vi "SP_OEE_2_test.vi"() -> ()   [LabVIEW 2017] (continued)
                      tunnel: [w17350] -> w17056
                      tunnel: [w17349] -> w17055
                      tunnel: [w17348] -> w17054
                      tunnel: [w17347] -> w17053
                      tunnel: [w17346] -> w17052
                      tunnel: [w17345] -> w17051
                      tunnel: [w17343] -> w17050
                      tunnel: [w17341] -> w17049
                      tunnel: [w17337] -> w17048
                      tunnel: [w17335] -> w17047
                      tunnel: w17062 -> [w17336]
                      tunnel: w17061 -> [w17332]
                      tunnel: [w17331] -> w17046
                      tunnel: w17060 -> [w17331]
                      tunnel: w17019 -> [w17329]
                      tunnel: w17059 -> [w17380]
                      tunnel: w17058 -> [w17373]
                      tunnel: w17057 -> [w17364]
                      tunnel: w17056 -> [w17372]
                      tunnel: w17055 -> [w17362]
                      tunnel: w17054 -> [w17371]
                      tunnel: w17053 -> [w17360]
                      tunnel: w17052 -> [w17370]
                      tunnel: w17051 -> [w17358]
                      tunnel: w17050 -> [w17394]
                      tunnel: w17049 -> [w17393]
                      tunnel: w17048 -> [w17369]
                      tunnel: w17047 -> [w17356]
                      tunnel: [w17394] -> w17045
                      tunnel: [w17393] -> w17044
                      tunnel: [w17387] -> w17043
                      tunnel: [w17380] -> w17042
                      tunnel: [w17379] -> w17041
                      tunnel: [w17378] -> w17040
                      tunnel: [w17377] -> w17039
                      tunnel: [w17376] -> w17038
                      tunnel: [w17375] -> w17037
                      tunnel: [w17374] -> w17036
                      tunnel: [w17373] -> w17035
                      tunnel: [w17372] -> w17034
                      tunnel: [w17371] -> w17033
                      tunnel: [w17370] -> w17032
                      tunnel: [w17369] -> w17031
                      tunnel: [w17354] -> w17030
                      tunnel: w17046 -> [w17354]
                      tunnel: [w17407] -> _
                      tunnel: [w17403] -> _
                      tunnel: w17045 -> [w17404]
                      tunnel: w17044 -> [w17407]
                      tunnel: w17043 -> [w17398]
                      tunnel: w17042 -> [w17405]
                      tunnel: w17041 -> [_]
                      tunnel: w17040 -> [_]
                      tunnel: w17039 -> [_]
                      tunnel: w17038 -> [_]
                      tunnel: w17037 -> [w17397]
                      tunnel: w17036 -> [w17399]
                      tunnel: w17035 -> [_]
                      tunnel: w17034 -> [_]
                      tunnel: w17033 -> [_]
                      tunnel: w17032 -> [_]
                      tunnel: w17031 -> [w17396]
                      tunnel: w17030 -> [w17402]
                      frame #0 {
                        w17134 = "%Y-%m-%d" ("time format string (%c)")
                        n3102 = Decimal String To Number(string=w17120) -> (number=w17121:i32)  [unwired: 2 in, 1 out]
                        n3103 = property on="Table" class="Tbl (strict)"("Visible"=TRUE) -> ()  [unwired: 2 in, 2 out]
                        n3104 = Format Date/Time String(time format string (%c)=w17134, seconds (now)=w17126) -> (date/time string=w17135:string)  [unwired: 1 in]
                        n3105 = Format Date/Time String(time format string (%c)=w17134, seconds (now)=w17125) -> (date/time string=w17133:string)  [unwired: 1 in]
                        n3106 = Format Into String(format string="Where BREAKDOWN_DATE between '%s' and '%s' and  SHIFT_ID = '%d'  ", w17135, w17133, w17121) -> (resulting string=w17132:string)  [unwired: 2 in, 1 out]
                        n3107 = call <vilib>:"DB Tools Select Data.vi"("condition"=w17132, "error in (no error)"=w17141, "columns"=string[] ["BREAKDOWN_DATE"], "table"="STATION_1_LOG_HISTORY", "connection reference"=w17143) -> ("error out"=w17128:errorcluster, "data"=w17131:variant[][], "connection reference out"=w17142:T2)  [unwired: 1 in]
                        n3108 = property on="Table 2" class="Tbl (strict)"("Visible"=FALSE) -> ()  [unwired: 2 in, 2 out]
                        n3109 = xnode "Database Variant To Data"("database variant"=w17131, "error in (no error)"=w17128, "type"=string[][] [] ("Elements Found")) -> ("data"=w17129:string[][], "error out"=w17127:errorcluster)
                        n3110 = Index Array(array=w17129, index (col)=0 ("disabled index (col)")) -> (element=w17137:string[])  [unwired: 1 in]
                        n3111 = call "Search_1d_array_element.vi"("Count in"=string[] [] ("Elements Found"), "BD Date"=w17137, "Elements Found in"=string[] [] ("Elements Found")) -> ("Elements Found out"=w17124:string[])  [unwired: 4 in, 2 out]
                        n3112 = Build Array(w17124) -> (w17147:string[][])
                        n3113 = Transpose 2D Array(2D array=w17147) -> (transposed array=w17146:string[][])
                      }
                      frame #1 {
                        n3114 = disable-structure shown="Enabled" {
                          disable-tunnel: w17209 -> [w17220 w17222]
                          disable-tunnel: [w17219 w17222] -> w17208
                          disable-tunnel: w17207 -> [w17218 w17223]
                          disable-tunnel: [w17217 w17223] -> w17206
                          disable-tunnel: w17204 -> [w17215 _]
                          disable-tunnel: w17203 -> [w17214 _]
                          disable-tunnel: [w17213 _] -> w17202
                          disable-tunnel: [w17212 _] -> w17199
                          disable-tunnel: w17197 -> [w17211 _]
                          disable-tunnel: w17194 -> [w17210 w17221]
                          disable-tunnel: [_ w17221] -> w17193
                          frame Disabled {
                            n3115 = call "Stack_holderwise_total_bd_count_&_duration_2.vi"("Refnum in"=w17220, "BREAKDOWN_STK_HOLD_ID"=1, "condition"=w17211, "Form Date"=w17215, "To Date"=w17214, "error in (no error)"=w17218, "Shift"=w17210) -> ("Refnum out"=w17219:T2, "Count out"=w17213:string[], "appended array"=w17212:dbl[], "error out"=w17217:errorcluster)  [unwired: 5 in]
                          }
                          frame Enabled {
                          }
                        }
                        n3116 = call "NUMERIC TO STRING.vi"("appended array"=w17199) -> ("Array"=w17198:string[])  [unwired: 4 in]
                        n3117 = call "Insert_empty_element_with_zero.vi"("searched date"=w17202, "fixed date"=w17200) -> ("O/P"=w17195:string[])  [unwired: 9 in]
                        n3118 = call "Insert_empty_element_with_zero.vi"("searched date"=w17198, "fixed date"=w17200) -> ("O/P"=w17201:string[])  [unwired: 9 in]
                      }
                      frame #2 {
                        n3119 = disable-structure shown="Enabled" {
                          disable-tunnel: w17239 -> [w17253 w17255]
                          disable-tunnel: [w17252 w17255] -> w17238
                          disable-tunnel: w17237 -> [w17251 w17256]
                          disable-tunnel: [w17250 w17256] -> w17236
                          disable-tunnel: w17235 -> [w17249 _]
                          disable-tunnel: w17234 -> [w17248 _]
                          disable-tunnel: [w17247 _] -> w17233
                          disable-tunnel: [w17246 _] -> w17229
                          disable-tunnel: w17227 -> [w17245 _]
                          disable-tunnel: w17225 -> [w17243 w17254]
                          disable-tunnel: [_ w17254] -> w17224
                          frame Disabled {
                            n3120 = call "Stack_holderwise_total_bd_count_&_duration_2.vi"("Refnum in"=w17251, "BREAKDOWN_STK_HOLD_ID"=2, "condition"=w17245, "Form Date"=w17249, "To Date"=w17248, "error in (no error)"=w17253, "Shift"=w17243) -> ("Refnum out"=w17250:T2, "Count out"=w17247:string[], "appended array"=w17246:dbl[], "error out"=w17252:errorcluster)  [unwired: 5 in]
                          }
                          frame Enabled {
                          }
                        }
                        n3121 = call "Insert_empty_element_with_zero.vi"("searched date"=w17233, "fixed date"=w17230) -> ("O/P"=w17232:string[])  [unwired: 9 in]
                        n3122 = call "NUMERIC TO STRING.vi"("appended array"=w17229) -> ("Array"=w17228:string[])  [unwired: 4 in]
                        n3123 = call "Insert_empty_element_with_zero.vi"("searched date"=w17228, "fixed date"=w17230) -> ("O/P"=w17231:string[])  [unwired: 9 in]
                      }
                      frame #3 {
                        n3124 = disable-structure shown="Enabled" {
                          disable-tunnel: w17272 -> [w17288 w17290]
                          disable-tunnel: [w17287 w17290] -> w17271
                          disable-tunnel: w17270 -> [w17286 w17291]
                          disable-tunnel: [w17285 w17291] -> w17269
                          disable-tunnel: w17268 -> [w17284 _]
                          disable-tunnel: w17267 -> [w17283 _]
                          disable-tunnel: [w17282 _] -> w17266
                          disable-tunnel: [w17281 _] -> w17262
                          disable-tunnel: w17260 -> [w17280 _]
                          disable-tunnel: w17258 -> [w17278 w17289]
                          disable-tunnel: [_ w17289] -> w17257
                          frame Disabled {
                            n3125 = call "Stack_holderwise_total_bd_count_&_duration_2.vi"("Refnum in"=w17286, "BREAKDOWN_STK_HOLD_ID"=3, "condition"=w17280, "Form Date"=w17284, "To Date"=w17283, "error in (no error)"=w17288, "Shift"=w17278) -> ("Refnum out"=w17285:T2, "Count out"=w17282:string[], "appended array"=w17281:dbl[], "error out"=w17287:errorcluster)  [unwired: 5 in]
                          }
                          frame Enabled {
                          }
                        }
                        n3126 = call "Insert_empty_element_with_zero.vi"("searched date"=w17266, "fixed date"=w17263) -> ("O/P"=w17265:string[])  [unwired: 9 in]
                        n3127 = call "NUMERIC TO STRING.vi"("appended array"=w17262) -> ("Array"=w17261:string[])  [unwired: 4 in]
                        n3128 = call "Insert_empty_element_with_zero.vi"("searched date"=w17261, "fixed date"=w17263) -> ("O/P"=w17264:string[])  [unwired: 9 in]
                      }
                      frame #4 {
                        n3129 = disable-structure shown="Enabled" {
                          disable-tunnel: w17307 -> [w17325 w17328]
                          disable-tunnel: w17306 -> [w17324 w17327]
                          disable-tunnel: [w17323 w17327] -> w17305
                          disable-tunnel: [w17322 w17328] -> w17304
                          disable-tunnel: w17303 -> [w17321 _]
                          disable-tunnel: w17302 -> [w17320 _]
                          disable-tunnel: [w17319 _] -> w17301
                          disable-tunnel: [w17318 _] -> w17297
                          disable-tunnel: w17295 -> [w17317 _]
                          disable-tunnel: w17293 -> [w17315 w17326]
                          disable-tunnel: [_ w17326] -> w17292
                          frame Disabled {
                            n3130 = call "Stack_holderwise_total_bd_count_&_duration_2.vi"("Refnum in"=w17324, "BREAKDOWN_STK_HOLD_ID"=4, "condition"=w17317, "Form Date"=w17321, "To Date"=w17320, "error in (no error)"=w17325, "Shift"=w17315) -> ("Refnum out"=w17323:T2, "Count out"=w17319:string[], "appended array"=w17318:dbl[], "error out"=w17322:errorcluster)  [unwired: 5 in]
                          }
                          frame Enabled {
                          }
                        }
                        n3131 = call "Insert_empty_element_with_zero.vi"("searched date"=w17301, "fixed date"=w17298) -> ("O/P"=w17300:string[])  [unwired: 9 in]
                        n3132 = call "NUMERIC TO STRING.vi"("appended array"=w17297) -> ("Array"=w17296:string[])  [unwired: 4 in]
                        n3133 = call "Insert_empty_element_with_zero.vi"("searched date"=w17296, "fixed date"=w17298) -> ("O/P"=w17299:string[])  [unwired: 9 in]
                      }
                      frame #5 {
                        n3134 = call "Stack_holderwise_total_bd_count_&_duration_2.vi"("Refnum in"=w17342, "BREAKDOWN_STK_HOLD_ID"=5, "condition"=w17332, "Form Date"=w17339, "To Date"=w17340, "error in (no error)"=w17344, "Shift"=w17329) -> ("Refnum out"=w17341:T2, "Count out"=w17338:string[], "appended array"=w17334:dbl[], "error out"=w17343:errorcluster)  [unwired: 5 in]
                        n3135 = call "NUMERIC TO STRING.vi"("appended array"=w17334) -> ("Array"=w17333:string[])  [unwired: 4 in]
                        n3136 = call "Insert_empty_element_with_zero.vi"("searched date"=w17338, "fixed date"=w17336) -> ("O/P"=w17337:string[])  [unwired: 9 in]
                        n3137 = call "Insert_empty_element_with_zero.vi"("searched date"=w17333, "fixed date"=w17336) -> ("O/P"=w17335:string[])  [unwired: 9 in]
                      }
                      frame #6 {
                        n3138 = call "String to numeric.vi"("Array"=w17364) -> ("Array 2"=w17363:dbl[])  [unwired: 4 in]
                        n3139 = call "String to numeric.vi"("Array"=w17362) -> ("Array 2"=w17361:dbl[])  [unwired: 4 in]
                        n3140 = call "String to numeric.vi"("Array"=w17360) -> ("Array 2"=w17359:dbl[])  [unwired: 4 in]
                        n3141 = call "String to numeric.vi"("Array"=w17358) -> ("Array 2"=w17357:dbl[])  [unwired: 4 in]
                        n3142 = call "String to numeric.vi"("Array"=w17356) -> ("Array 2"=w17355:dbl[])  [unwired: 4 in]
                        n3143 = Decimal String To Number(string=w17369) -> (number=w17388:i32[])  [unwired: 2 in, 1 out]
                        n3144 = Decimal String To Number(string=w17370) -> (number=w17389:i32[])  [unwired: 2 in, 1 out]
                        n3145 = Decimal String To Number(string=w17371) -> (number=w17390:i32[])  [unwired: 2 in, 1 out]
                        n3146 = Decimal String To Number(string=w17372) -> (number=w17391:i32[])  [unwired: 2 in, 1 out]
                        n3147 = Decimal String To Number(string=w17373) -> (number=w17386:i32[])  [unwired: 2 in, 1 out]
                        n3148 = Compound Arithmetic op=ADD(w17363, w17361, w17359, w17357, w17355) -> (w17366:dbl[])
                        n3149 = Build Array(w17364) -> (w17385:string[][])
                        n3150 = Build Array(w17362) -> (w17384:string[][])
                        n3151 = Build Array(w17360) -> (w17383:string[][])
                        n3152 = Build Array(w17358) -> (w17382:string[][])
                        n3153 = Build Array(w17356) -> (w17381:string[][])
                        n3154 = Number To Fractional String(number=w17366, precision (6)=i16 2) -> (F-format string=w17365:string[])  [unwired: 2 in]
                        n3155 = Compound Arithmetic op=ADD(w17388, w17389, w17390, w17391, w17386) -> (w17392:i32[])
                        n3156 = Transpose 2D Array(2D array=w17385) -> (transposed array=w17379:string[][])
                        n3157 = Transpose 2D Array(2D array=w17384) -> (transposed array=w17378:string[][])
                        n3158 = Transpose 2D Array(2D array=w17383) -> (transposed array=w17377:string[][])
                        n3159 = Transpose 2D Array(2D array=w17382) -> (transposed array=w17376:string[][])
                        n3160 = Transpose 2D Array(2D array=w17381) -> (transposed array=w17375:string[][])
                        n3161 = Number To Decimal String(number=w17392) -> (decimal integer string=w17387:string[])  [unwired: 1 in]
                        n3162 = Build Array(w17365) -> (w17368:string[][])
                        n3163 = Transpose 2D Array(2D array=w17368) -> (transposed array=w17374:string[][])
                      }
                      frame #7 {
                        w17395 = string[] [""]
                        n3164 = Insert Into Array(array=w17405, index (col)=1 ("disabled index (col)"), new element #1=w17395, new element #2=w17395, new element #3=w17395, new element #4=w17395, new element #5=w17395, new element #6=w17395, new element #7=w17395, new element #8=w17395, new element #9=w17396, new element #10=w17397, new element #11=w17398, new element #12=w17399) -> (w17401:string[][])  [unwired: 1 in]
                        n3165 = call "flot graph for month n year.vi"("BD Date"=w17402, "error in (no error)"=w17404, "Count total"=w17398) -> ("error out"=w17403:errorcluster, "Run-Time Status"=w17400:cluster{"Array 2":timestamp[], dbl[]})  [unwired: 7 in]
                        n3166 = local write "Run-Time Status"(w17400) -> ()
                        n3167 = local write "Table"(w17401) -> ()
                      }
                    }
                  }
                  frame "1" {
                    n3168 = flat-sequence {
                      tunnel: w17418 -> [w17532]
                      tunnel: w17417 -> [w17530]
                      tunnel: [w17516] -> w17508
                      tunnel: [w17531] -> w17507
                      tunnel: w17416 -> [_]
                      tunnel: [w17535] -> w17506
                      tunnel: [w17515] -> w17505
                      tunnel: [w17514] -> w17504
                      tunnel: [w17513] -> w17503
                      tunnel: w17415 -> [w17515]
                      tunnel: w17414 -> [w17514]
                      tunnel: ["Where BREAKDOWN_DATE between '%s'and '%s' and BREAKDOWN_STK_HOLD_ID ='%d' and  SHIFT_ID = '%d' "] -> w17502
                      tunnel: [w17513] -> w17501
                      tunnel: w17413 -> [w17509]
                      tunnel: [w17509] -> w17412
                      tunnel: w17508 -> [w17596]
                      tunnel: w17507 -> [w17598]
                      tunnel: w17506 -> [w17594]
                      tunnel: w17505 -> [w17593]
                      tunnel: w17504 -> [w17592]
                      tunnel: [w17595] -> w17500
                      tunnel: [w17597] -> w17499
                      tunnel: [w17594] -> w17498
                      tunnel: [w17584] -> w17497
                      tunnel: [w17590] -> w17496
                      tunnel: [w17593] -> w17495
                      tunnel: [w17592] -> w17494
                      tunnel: w17503 -> [w17589]
                      tunnel: [w17589] -> w17493
                      tunnel: w17502 -> [w17586]
                      tunnel: [w17586] -> w17492
                      tunnel: [w17585] -> w17491
                      tunnel: w17501 -> [w17585]
                      tunnel: w17412 -> [w17583]
                      tunnel: [w17582] -> w17411
                      tunnel: w17500 -> [w17628]
                      tunnel: w17499 -> [w17626]
                      tunnel: w17498 -> [w17631]
                      tunnel: w17497 -> [w17630]
                      tunnel: w17496 -> [w17629]
                      tunnel: w17495 -> [w17624]
                      tunnel: w17494 -> [w17623]
                      tunnel: [w17631] -> w17490
                      tunnel: [w17630] -> w17489
                      tunnel: [w17629] -> w17488
                      tunnel: [w17627] -> w17487
                      tunnel: [w17621] -> w17486
                      tunnel: [w17620] -> w17485
                      tunnel: [w17625] -> w17484
                      tunnel: [w17624] -> w17483
                      tunnel: [w17623] -> w17482
                      tunnel: w17493 -> [w17619]
                      tunnel: [w17619] -> w17481
                      tunnel: w17492 -> [w17616]
                      tunnel: [w17616] -> w17480
                      tunnel: [w17615] -> w17479
                      tunnel: w17491 -> [w17615]
                      tunnel: w17411 -> [w17614]
                      tunnel: [w17613] -> w17410
                      tunnel: w17490 -> [w17666]
                      tunnel: w17489 -> [w17665]
                      tunnel: w17488 -> [w17664]
                      tunnel: w17487 -> [w17661]
                      tunnel: w17486 -> [w17663]
                      tunnel: w17485 -> [w17662]
                      tunnel: w17484 -> [w17659]
                      tunnel: w17483 -> [w17657]
                      tunnel: w17482 -> [w17656]
                      tunnel: [w17666] -> w17478
                      tunnel: [w17665] -> w17477
                      tunnel: [w17664] -> w17476
                      tunnel: [w17663] -> w17475
                      tunnel: [w17662] -> w17474
                      tunnel: [w17660] -> w17473
                      tunnel: [w17654] -> w17472
                      tunnel: [w17653] -> w17471
                      tunnel: [w17658] -> w17470
                      tunnel: [w17657] -> w17469
                      tunnel: [w17656] -> w17468
                      tunnel: w17481 -> [w17652]
                      tunnel: [w17652] -> w17467
                      tunnel: w17480 -> [w17649]
                      tunnel: [w17649] -> w17466
                      tunnel: [w17648] -> w17465
                      tunnel: w17479 -> [w17648]
                      tunnel: w17410 -> [w17647]
                      tunnel: [w17646] -> w17409
                      tunnel: w17478 -> [w17703]
                      tunnel: w17477 -> [w17702]
                      tunnel: w17476 -> [w17701]
                      tunnel: w17475 -> [w17700]
                      tunnel: w17474 -> [w17699]
                      tunnel: w17473 -> [w17696]
                      tunnel: w17472 -> [w17698]
                      tunnel: w17471 -> [w17697]
                      tunnel: w17470 -> [w17695]
                      tunnel: w17469 -> [w17692]
                      tunnel: w17468 -> [w17691]
                      tunnel: [w17703] -> w17464
                      tunnel: [w17702] -> w17463
                      tunnel: [w17701] -> w17462
                      tunnel: [w17700] -> w17461
                      tunnel: [w17699] -> w17460
                      tunnel: [w17698] -> w17459
                      tunnel: [w17697] -> w17458
                      tunnel: [w17694] -> w17457
                      tunnel: [w17693] -> w17456
                      tunnel: [w17689] -> w17455
                      tunnel: [w17688] -> w17454
                      tunnel: [w17692] -> w17453
                      tunnel: [w17691] -> w17452
                      tunnel: w17467 -> [w17687]
                      tunnel: [w17687] -> w17451
                      tunnel: w17466 -> [w17684]
                      tunnel: [w17684] -> w17450
                      tunnel: [w17683] -> w17449
                      tunnel: w17465 -> [w17683]
                      tunnel: w17409 -> [w17682]
                      tunnel: [w17681] -> w17408
                      tunnel: w17464 -> [w17742]
                      tunnel: w17463 -> [w17741]
                      tunnel: w17462 -> [w17740]
                      tunnel: w17461 -> [w17739]
                      tunnel: w17460 -> [w17738]
                      tunnel: w17459 -> [w17737]
                      tunnel: w17458 -> [w17736]
                      tunnel: w17457 -> [w17731]
                      tunnel: w17456 -> [w17733]
                      tunnel: w17455 -> [w17735]
                      tunnel: w17454 -> [w17734]
                      tunnel: w17453 -> [w17728]
                      tunnel: w17452 -> [w17729]
                      tunnel: [w17742] -> w17448
                      tunnel: [w17741] -> w17447
                      tunnel: [w17740] -> w17446
                      tunnel: [w17739] -> w17445
                      tunnel: [w17738] -> w17444
                      tunnel: [w17737] -> w17443
                      tunnel: [w17736] -> w17442
                      tunnel: [w17735] -> w17441
                      tunnel: [w17734] -> w17440
                      tunnel: [w17732] -> w17439
                      tunnel: [w17730] -> w17438
                      tunnel: [w17726] -> w17437
                      tunnel: [w17724] -> w17436
                      tunnel: w17451 -> [w17725]
                      tunnel: w17450 -> [w17721]
                      tunnel: [w17720] -> w17435
                      tunnel: w17449 -> [w17720]
                      tunnel: w17408 -> [w17718]
                      tunnel: w17448 -> [w17769]
                      tunnel: w17447 -> [w17762]
                      tunnel: w17446 -> [w17753]
                      tunnel: w17445 -> [w17761]
                      tunnel: w17444 -> [w17751]
                      tunnel: w17443 -> [w17760]
                      tunnel: w17442 -> [w17749]
                      tunnel: w17441 -> [w17759]
                      tunnel: w17440 -> [w17747]
                      tunnel: w17439 -> [w17783]
                      tunnel: w17438 -> [w17782]
                      tunnel: w17437 -> [w17758]
                      tunnel: w17436 -> [w17745]
                      tunnel: [w17783] -> w17434
                      tunnel: [w17782] -> w17433
                      tunnel: [w17776] -> w17432
                      tunnel: [w17769] -> w17431
                      tunnel: [w17768] -> w17430
                      tunnel: [w17767] -> w17429
                      tunnel: [w17766] -> w17428
                      tunnel: [w17765] -> w17427
                      tunnel: [w17764] -> w17426
                      tunnel: [w17763] -> w17425
                      tunnel: [w17762] -> w17424
                      tunnel: [w17761] -> w17423
                      tunnel: [w17760] -> w17422
                      tunnel: [w17759] -> w17421
                      tunnel: [w17758] -> w17420
                      tunnel: [w17743] -> w17419
                      tunnel: w17435 -> [w17743]
                      tunnel: [w17796] -> _
                      tunnel: [w17792] -> _
                      tunnel: w17434 -> [w17793]
                      tunnel: w17433 -> [w17796]
                      tunnel: w17432 -> [w17787]
                      tunnel: w17431 -> [w17794]
                      tunnel: w17430 -> [_]
                      tunnel: w17429 -> [_]
                      tunnel: w17428 -> [_]
                      tunnel: w17427 -> [_]
                      tunnel: w17426 -> [w17786]
                      tunnel: w17425 -> [w17788]
                      tunnel: w17424 -> [_]
                      tunnel: w17423 -> [_]
                      tunnel: w17422 -> [_]
                      tunnel: w17421 -> [_]
                      tunnel: w17420 -> [w17785]
                      tunnel: w17419 -> [w17791]
                      frame #0 {
                        w17523 = "%Y-%m-%d" ("time format string (%c)")
                        n3169 = Decimal String To Number(string=w17509) -> (number=w17510:i32)  [unwired: 2 in, 1 out]
                        n3170 = property on="Table" class="Tbl (strict)"("Visible"=TRUE) -> ()  [unwired: 2 in, 2 out]
                        n3171 = Format Date/Time String(time format string (%c)=w17523, seconds (now)=w17515) -> (date/time string=w17524:string)  [unwired: 1 in]
                        n3172 = Format Date/Time String(time format string (%c)=w17523, seconds (now)=w17514) -> (date/time string=w17522:string)  [unwired: 1 in]
                        n3173 = Format Into String(format string="Where BREAKDOWN_DATE between '%s' and '%s' and  SHIFT_ID = '%d'  ", w17524, w17522, w17510) -> (resulting string=w17521:string)  [unwired: 2 in, 1 out]
                        n3174 = call <vilib>:"DB Tools Select Data.vi"("condition"=w17521, "error in (no error)"=w17530, "columns"=string[] ["BREAKDOWN_DATE"], "table"="STATION_1_LOG_HISTORY", "connection reference"=w17532) -> ("error out"=w17517:errorcluster, "data"=w17520:variant[][], "connection reference out"=w17531:T2)  [unwired: 1 in]
                        n3175 = property on="Table 2" class="Tbl (strict)"("Visible"=FALSE) -> ()  [unwired: 2 in, 2 out]
                        n3176 = xnode "Database Variant To Data"("database variant"=w17520, "error in (no error)"=w17517, "type"=string[][] [] ("Elements Found")) -> ("data"=w17518:string[][], "error out"=w17516:errorcluster)
                        n3177 = Index Array(array=w17518, index (col)=0 ("disabled index (col)")) -> (element=w17526:string[])  [unwired: 1 in]
                        n3178 = call "Search_1d_array_element.vi"("Count in"=string[] [] ("Elements Found"), "BD Date"=w17526, "Elements Found in"=string[] [] ("Elements Found")) -> ("Elements Found out"=w17513:string[])  [unwired: 4 in, 2 out]
                        n3179 = Build Array(w17513) -> (w17536:string[][])
                        n3180 = Transpose 2D Array(2D array=w17536) -> (transposed array=w17535:string[][])
                      }
                      frame #1 {
                        n3181 = disable-structure shown="Enabled" {
                          disable-tunnel: w17598 -> [w17609 w17611]
                          disable-tunnel: [w17608 w17611] -> w17597
                          disable-tunnel: w17596 -> [w17607 w17612]
                          disable-tunnel: [w17606 w17612] -> w17595
                          disable-tunnel: w17593 -> [w17604 _]
                          disable-tunnel: w17592 -> [w17603 _]
                          disable-tunnel: [w17602 _] -> w17591
                          disable-tunnel: [w17601 _] -> w17588
                          disable-tunnel: w17586 -> [w17600 _]
                          disable-tunnel: w17583 -> [w17599 w17610]
                          disable-tunnel: [_ w17610] -> w17582
                          frame Disabled {
                            n3182 = call "Stack_holderwise_total_bd_count_&_duration_2.vi"("Refnum in"=w17609, "BREAKDOWN_STK_HOLD_ID"=1, "condition"=w17600, "Form Date"=w17604, "To Date"=w17603, "error in (no error)"=w17607, "Shift"=w17599) -> ("Refnum out"=w17608:T2, "Count out"=w17602:string[], "appended array"=w17601:dbl[], "error out"=w17606:errorcluster)  [unwired: 5 in]
                          }
                          frame Enabled {
                          }
                        }
                        n3183 = call "NUMERIC TO STRING.vi"("appended array"=w17588) -> ("Array"=w17587:string[])  [unwired: 4 in]
                        n3184 = call "Insert_empty_element_with_zero.vi"("searched date"=w17591, "fixed date"=w17589) -> ("O/P"=w17584:string[])  [unwired: 9 in]
                        n3185 = call "Insert_empty_element_with_zero.vi"("searched date"=w17587, "fixed date"=w17589) -> ("O/P"=w17590:string[])  [unwired: 9 in]
                      }
                      frame #2 {
                        n3186 = disable-structure shown="Enabled" {
                          disable-tunnel: w17628 -> [w17642 w17644]
                          disable-tunnel: [w17641 w17644] -> w17627
                          disable-tunnel: w17626 -> [w17640 w17645]
                          disable-tunnel: [w17639 w17645] -> w17625
                          disable-tunnel: w17624 -> [w17638 _]
                          disable-tunnel: w17623 -> [w17637 _]
                          disable-tunnel: [w17636 _] -> w17622
                          disable-tunnel: [w17635 _] -> w17618
                          disable-tunnel: w17616 -> [w17634 _]
                          disable-tunnel: w17614 -> [w17632 w17643]
                          disable-tunnel: [_ w17643] -> w17613
                          frame Disabled {
                            n3187 = call "Stack_holderwise_total_bd_count_&_duration_2.vi"("Refnum in"=w17640, "BREAKDOWN_STK_HOLD_ID"=2, "condition"=w17634, "Form Date"=w17638, "To Date"=w17637, "error in (no error)"=w17642, "Shift"=w17632) -> ("Refnum out"=w17639:T2, "Count out"=w17636:string[], "appended array"=w17635:dbl[], "error out"=w17641:errorcluster)  [unwired: 5 in]
                          }
                          frame Enabled {
                          }
                        }
                        n3188 = call "Insert_empty_element_with_zero.vi"("searched date"=w17622, "fixed date"=w17619) -> ("O/P"=w17621:string[])  [unwired: 9 in]
                        n3189 = call "NUMERIC TO STRING.vi"("appended array"=w17618) -> ("Array"=w17617:string[])  [unwired: 4 in]
                        n3190 = call "Insert_empty_element_with_zero.vi"("searched date"=w17617, "fixed date"=w17619) -> ("O/P"=w17620:string[])  [unwired: 9 in]
                      }
                      frame #3 {
                        n3191 = disable-structure shown="Enabled" {
                          disable-tunnel: w17661 -> [w17677 w17679]
                          disable-tunnel: [w17676 w17679] -> w17660
                          disable-tunnel: w17659 -> [w17675 w17680]
                          disable-tunnel: [w17674 w17680] -> w17658
                          disable-tunnel: w17657 -> [w17673 _]
                          disable-tunnel: w17656 -> [w17672 _]
                          disable-tunnel: [w17671 _] -> w17655
                          disable-tunnel: [w17670 _] -> w17651
                          disable-tunnel: w17649 -> [w17669 _]
                          disable-tunnel: w17647 -> [w17667 w17678]
                          disable-tunnel: [_ w17678] -> w17646
                          frame Disabled {
                            n3192 = call "Stack_holderwise_total_bd_count_&_duration_2.vi"("Refnum in"=w17675, "BREAKDOWN_STK_HOLD_ID"=3, "condition"=w17669, "Form Date"=w17673, "To Date"=w17672, "error in (no error)"=w17677, "Shift"=w17667) -> ("Refnum out"=w17674:T2, "Count out"=w17671:string[], "appended array"=w17670:dbl[], "error out"=w17676:errorcluster)  [unwired: 5 in]
                          }
                          frame Enabled {
                          }
                        }
                        n3193 = call "Insert_empty_element_with_zero.vi"("searched date"=w17655, "fixed date"=w17652) -> ("O/P"=w17654:string[])  [unwired: 9 in]
                        n3194 = call "NUMERIC TO STRING.vi"("appended array"=w17651) -> ("Array"=w17650:string[])  [unwired: 4 in]
                        n3195 = call "Insert_empty_element_with_zero.vi"("searched date"=w17650, "fixed date"=w17652) -> ("O/P"=w17653:string[])  [unwired: 9 in]
                      }
                      frame #4 {
                        n3196 = disable-structure shown="Enabled" {
                          disable-tunnel: w17696 -> [w17714 w17717]
                          disable-tunnel: w17695 -> [w17713 w17716]
                          disable-tunnel: [w17712 w17716] -> w17694
                          disable-tunnel: [w17711 w17717] -> w17693
                          disable-tunnel: w17692 -> [w17710 _]
                          disable-tunnel: w17691 -> [w17709 _]
                          disable-tunnel: [w17708 _] -> w17690
                          disable-tunnel: [w17707 _] -> w17686
                          disable-tunnel: w17684 -> [w17706 _]
                          disable-tunnel: w17682 -> [w17704 w17715]
                          disable-tunnel: [_ w17715] -> w17681
                          frame Disabled {
                            n3197 = call "Stack_holderwise_total_bd_count_&_duration_2.vi"("Refnum in"=w17713, "BREAKDOWN_STK_HOLD_ID"=4, "condition"=w17706, "Form Date"=w17710, "To Date"=w17709, "error in (no error)"=w17714, "Shift"=w17704) -> ("Refnum out"=w17712:T2, "Count out"=w17708:string[], "appended array"=w17707:dbl[], "error out"=w17711:errorcluster)  [unwired: 5 in]
                          }
                          frame Enabled {
                          }
                        }
                        n3198 = call "Insert_empty_element_with_zero.vi"("searched date"=w17690, "fixed date"=w17687) -> ("O/P"=w17689:string[])  [unwired: 9 in]
                        n3199 = call "NUMERIC TO STRING.vi"("appended array"=w17686) -> ("Array"=w17685:string[])  [unwired: 4 in]
                        n3200 = call "Insert_empty_element_with_zero.vi"("searched date"=w17685, "fixed date"=w17687) -> ("O/P"=w17688:string[])  [unwired: 9 in]
                      }
                      frame #5 {
                        n3201 = call "Stack_holderwise_total_bd_count_&_duration_2.vi"("Refnum in"=w17731, "BREAKDOWN_STK_HOLD_ID"=5, "condition"=w17721, "Form Date"=w17728, "To Date"=w17729, "error in (no error)"=w17733, "Shift"=w17718) -> ("Refnum out"=w17730:T2, "Count out"=w17727:string[], "appended array"=w17723:dbl[], "error out"=w17732:errorcluster)  [unwired: 5 in]
                        n3202 = call "NUMERIC TO STRING.vi"("appended array"=w17723) -> ("Array"=w17722:string[])  [unwired: 4 in]
                        n3203 = call "Insert_empty_element_with_zero.vi"("searched date"=w17727, "fixed date"=w17725) -> ("O/P"=w17726:string[])  [unwired: 9 in]
                        n3204 = call "Insert_empty_element_with_zero.vi"("searched date"=w17722, "fixed date"=w17725) -> ("O/P"=w17724:string[])  [unwired: 9 in]
                      }
                      frame #6 {
                        n3205 = call "String to numeric.vi"("Array"=w17753) -> ("Array 2"=w17752:dbl[])  [unwired: 4 in]
                        n3206 = call "String to numeric.vi"("Array"=w17751) -> ("Array 2"=w17750:dbl[])  [unwired: 4 in]
                        n3207 = call "String to numeric.vi"("Array"=w17749) -> ("Array 2"=w17748:dbl[])  [unwired: 4 in]
                        n3208 = call "String to numeric.vi"("Array"=w17747) -> ("Array 2"=w17746:dbl[])  [unwired: 4 in]
                        n3209 = call "String to numeric.vi"("Array"=w17745) -> ("Array 2"=w17744:dbl[])  [unwired: 4 in]
                        n3210 = Decimal String To Number(string=w17758) -> (number=w17777:i32[])  [unwired: 2 in, 1 out]
                        n3211 = Decimal String To Number(string=w17759) -> (number=w17778:i32[])  [unwired: 2 in, 1 out]
                        n3212 = Decimal String To Number(string=w17760) -> (number=w17779:i32[])  [unwired: 2 in, 1 out]
                        n3213 = Decimal String To Number(string=w17761) -> (number=w17780:i32[])  [unwired: 2 in, 1 out]
                        n3214 = Decimal String To Number(string=w17762) -> (number=w17775:i32[])  [unwired: 2 in, 1 out]
                        n3215 = Compound Arithmetic op=ADD(w17752, w17750, w17748, w17746, w17744) -> (w17755:dbl[])
                        n3216 = Build Array(w17753) -> (w17774:string[][])
                        n3217 = Build Array(w17751) -> (w17773:string[][])
                        n3218 = Build Array(w17749) -> (w17772:string[][])
                        n3219 = Build Array(w17747) -> (w17771:string[][])
                        n3220 = Build Array(w17745) -> (w17770:string[][])
                        n3221 = Number To Fractional String(number=w17755, precision (6)=i16 2) -> (F-format string=w17754:string[])  [unwired: 2 in]
                        n3222 = Compound Arithmetic op=ADD(w17777, w17778, w17779, w17780, w17775) -> (w17781:i32[])
                        n3223 = Transpose 2D Array(2D array=w17774) -> (transposed array=w17768:string[][])
                        n3224 = Transpose 2D Array(2D array=w17773) -> (transposed array=w17767:string[][])
                        n3225 = Transpose 2D Array(2D array=w17772) -> (transposed array=w17766:string[][])
                        n3226 = Transpose 2D Array(2D array=w17771) -> (transposed array=w17765:string[][])
                        n3227 = Transpose 2D Array(2D array=w17770) -> (transposed array=w17764:string[][])
                        n3228 = Number To Decimal String(number=w17781) -> (decimal integer string=w17776:string[])  [unwired: 1 in]
                        n3229 = Build Array(w17754) -> (w17757:string[][])
                        n3230 = Transpose 2D Array(2D array=w17757) -> (transposed array=w17763:string[][])
                      }
                      frame #7 {
                        w17784 = string[] [""]
                        n3231 = Insert Into Array(array=w17794, index (col)=1 ("disabled index (col)"), new element #1=w17784, new element #2=w17784, new element #3=w17784, new element #4=w17784, new element #5=w17784, new element #6=w17784, new element #7=w17784, new element #8=w17784, new element #9=w17785, new element #10=w17786, new element #11=w17787, new element #12=w17788) -> (w17790:string[][])  [unwired: 1 in]
                        n3232 = call "flot graph for month n year.vi"("BD Date"=w17791, "error in (no error)"=w17793, "Count total"=w17787) -> ("error out"=w17792:errorcluster, "Run-Time Status"=w17789:cluster{"Array 2":timestamp[], dbl[]})  [unwired: 7 in]
                        n3233 = local write "Run-Time Status"(w17789) -> ()
                        n3234 = local write "Table"(w17790) -> ()
                      }
                    }
                  }
                  frame "2" {
                    n3235 = flat-sequence {
                      tunnel: w17807 -> [w17921]
                      tunnel: w17806 -> [w17919]
                      tunnel: [w17905] -> w17897
                      tunnel: [w17920] -> w17896
                      tunnel: w17805 -> [_]
                      tunnel: [w17924] -> w17895
                      tunnel: [w17904] -> w17894
                      tunnel: [w17903] -> w17893
                      tunnel: [w17902] -> w17892
                      tunnel: w17804 -> [w17904]
                      tunnel: w17803 -> [w17903]
                      tunnel: ["Where BREAKDOWN_DATE between '%s'and '%s' and BREAKDOWN_STK_HOLD_ID ='%d' and  SHIFT_ID = '%d' "] -> w17891
                      tunnel: [w17902] -> w17890
                      tunnel: w17802 -> [w17898]
                      tunnel: [w17898] -> w17801
                      tunnel: w17897 -> [w17985]
                      tunnel: w17896 -> [w17987]
                      tunnel: w17895 -> [w17983]
                      tunnel: w17894 -> [w17982]
                      tunnel: w17893 -> [w17981]
                      tunnel: [w17984] -> w17889
                      tunnel: [w17986] -> w17888
                      tunnel: [w17983] -> w17887
                      tunnel: [w17973] -> w17886
                      tunnel: [w17979] -> w17885
                      tunnel: [w17982] -> w17884
                      tunnel: [w17981] -> w17883
                      tunnel: w17892 -> [w17978]
                      tunnel: [w17978] -> w17882
                      tunnel: w17891 -> [w17975]
                      tunnel: [w17975] -> w17881
                      tunnel: [w17974] -> w17880
                      tunnel: w17890 -> [w17974]
                      tunnel: w17801 -> [w17972]
                      tunnel: [w17971] -> w17800
                      tunnel: w17889 -> [w18017]
                      tunnel: w17888 -> [w18015]
                      tunnel: w17887 -> [w18020]
                      tunnel: w17886 -> [w18019]
                      tunnel: w17885 -> [w18018]
                      tunnel: w17884 -> [w18013]
                      tunnel: w17883 -> [w18012]
                      tunnel: [w18020] -> w17879
                      tunnel: [w18019] -> w17878
                      tunnel: [w18018] -> w17877
                      tunnel: [w18016] -> w17876
                      tunnel: [w18010] -> w17875
                      tunnel: [w18009] -> w17874
                      tunnel: [w18014] -> w17873
                      tunnel: [w18013] -> w17872
                      tunnel: [w18012] -> w17871
                      tunnel: w17882 -> [w18008]
                      tunnel: [w18008] -> w17870
                      tunnel: w17881 -> [w18005]
                      tunnel: [w18005] -> w17869
                      tunnel: [w18004] -> w17868
                      tunnel: w17880 -> [w18004]
                      tunnel: w17800 -> [w18003]
                      tunnel: [w18002] -> w17799
                      tunnel: w17879 -> [w18055]
                      tunnel: w17878 -> [w18054]
                      tunnel: w17877 -> [w18053]
                      tunnel: w17876 -> [w18050]
                      tunnel: w17875 -> [w18052]
                      tunnel: w17874 -> [w18051]
                      tunnel: w17873 -> [w18048]
                      tunnel: w17872 -> [w18046]
                      tunnel: w17871 -> [w18045]
                      tunnel: [w18055] -> w17867
                      tunnel: [w18054] -> w17866
                      tunnel: [w18053] -> w17865
                      tunnel: [w18052] -> w17864
                      tunnel: [w18051] -> w17863
                      tunnel: [w18049] -> w17862
                      tunnel: [w18043] -> w17861
                      tunnel: [w18042] -> w17860
                      tunnel: [w18047] -> w17859
                      tunnel: [w18046] -> w17858
                      tunnel: [w18045] -> w17857
                      tunnel: w17870 -> [w18041]
                      tunnel: [w18041] -> w17856
                      tunnel: w17869 -> [w18038]
                      tunnel: [w18038] -> w17855
                      tunnel: [w18037] -> w17854
                      tunnel: w17868 -> [w18037]
                      tunnel: w17799 -> [w18036]
                      tunnel: [w18035] -> w17798
                      tunnel: w17867 -> [w18092]
                      tunnel: w17866 -> [w18091]
                      tunnel: w17865 -> [w18090]
                      tunnel: w17864 -> [w18089]
                      tunnel: w17863 -> [w18088]
                      tunnel: w17862 -> [w18085]
                      tunnel: w17861 -> [w18087]
                      tunnel: w17860 -> [w18086]
                      tunnel: w17859 -> [w18084]
                      tunnel: w17858 -> [w18081]
                      tunnel: w17857 -> [w18080]
                      tunnel: [w18092] -> w17853
                      tunnel: [w18091] -> w17852
                      tunnel: [w18090] -> w17851
                      tunnel: [w18089] -> w17850
                      tunnel: [w18088] -> w17849
                      tunnel: [w18087] -> w17848
                      tunnel: [w18086] -> w17847
                      tunnel: [w18083] -> w17846
                      tunnel: [w18082] -> w17845
                      tunnel: [w18078] -> w17844
                      tunnel: [w18077] -> w17843
                      tunnel: [w18081] -> w17842
                      tunnel: [w18080] -> w17841
                      tunnel: w17856 -> [w18076]
                      tunnel: [w18076] -> w17840
                      tunnel: w17855 -> [w18073]
                      tunnel: [w18073] -> w17839
                      tunnel: [w18072] -> w17838
                      tunnel: w17854 -> [w18072]
                      tunnel: w17798 -> [w18071]
                      tunnel: [w18070] -> w17797
                      tunnel: w17853 -> [w18131]
                      tunnel: w17852 -> [w18130]
                      tunnel: w17851 -> [w18129]
                      tunnel: w17850 -> [w18128]
                      tunnel: w17849 -> [w18127]
                      tunnel: w17848 -> [w18126]
                      tunnel: w17847 -> [w18125]
                      tunnel: w17846 -> [w18120]
                      tunnel: w17845 -> [w18122]
                      tunnel: w17844 -> [w18124]
                      tunnel: w17843 -> [w18123]
                      tunnel: w17842 -> [w18117]
                      tunnel: w17841 -> [w18118]
                      tunnel: [w18131] -> w17837
                      tunnel: [w18130] -> w17836
                      tunnel: [w18129] -> w17835
                      tunnel: [w18128] -> w17834
                      tunnel: [w18127] -> w17833
                      tunnel: [w18126] -> w17832
                      tunnel: [w18125] -> w17831
                      tunnel: [w18124] -> w17830
                      tunnel: [w18123] -> w17829
                      tunnel: [w18121] -> w17828
                      tunnel: [w18119] -> w17827
                      tunnel: [w18115] -> w17826
                      tunnel: [w18113] -> w17825
                      tunnel: w17840 -> [w18114]
                      tunnel: w17839 -> [w18110]
                      tunnel: [w18109] -> w17824
                      tunnel: w17838 -> [w18109]
                      tunnel: w17797 -> [w18107]
                      tunnel: w17837 -> [w18158]
                      tunnel: w17836 -> [w18151]
                      tunnel: w17835 -> [w18142]
                      tunnel: w17834 -> [w18150]
                      tunnel: w17833 -> [w18140]
                      tunnel: w17832 -> [w18149]
                      tunnel: w17831 -> [w18138]
                      tunnel: w17830 -> [w18148]
                      tunnel: w17829 -> [w18136]
                      tunnel: w17828 -> [w18172]
                      tunnel: w17827 -> [w18171]
                      tunnel: w17826 -> [w18147]
                      tunnel: w17825 -> [w18134]
                      tunnel: [w18172] -> w17823
                      tunnel: [w18171] -> w17822
                      tunnel: [w18165] -> w17821
                      tunnel: [w18158] -> w17820
                      tunnel: [w18157] -> w17819
                      tunnel: [w18156] -> w17818
                      tunnel: [w18155] -> w17817
                      tunnel: [w18154] -> w17816
                      tunnel: [w18153] -> w17815
                      tunnel: [w18152] -> w17814
                      tunnel: [w18151] -> w17813
                      tunnel: [w18150] -> w17812
                      tunnel: [w18149] -> w17811
                      tunnel: [w18148] -> w17810
                      tunnel: [w18147] -> w17809
                      tunnel: [w18132] -> w17808
                      tunnel: w17824 -> [w18132]
                      tunnel: [w18185] -> _
                      tunnel: [w18181] -> _
                      tunnel: w17823 -> [w18182]
                      tunnel: w17822 -> [w18185]
                      tunnel: w17821 -> [w18176]
                      tunnel: w17820 -> [w18183]
                      tunnel: w17819 -> [_]
                      tunnel: w17818 -> [_]
                      tunnel: w17817 -> [_]
                      tunnel: w17816 -> [_]
                      tunnel: w17815 -> [w18175]
                      tunnel: w17814 -> [w18177]
                      tunnel: w17813 -> [_]
                      tunnel: w17812 -> [_]
                      tunnel: w17811 -> [_]
                      tunnel: w17810 -> [_]
                      tunnel: w17809 -> [w18174]
                      tunnel: w17808 -> [w18180]
                      frame #0 {
                        w17912 = "%Y-%m-%d" ("time format string (%c)")
                        n3236 = Decimal String To Number(string=w17898) -> (number=w17899:i32)  [unwired: 2 in, 1 out]
                        n3237 = property on="Table" class="Tbl (strict)"("Visible"=TRUE) -> ()  [unwired: 2 in, 2 out]
                        n3238 = Format Date/Time String(time format string (%c)=w17912, seconds (now)=w17904) -> (date/time string=w17913:string)  [unwired: 1 in]
                        n3239 = Format Date/Time String(time format string (%c)=w17912, seconds (now)=w17903) -> (date/time string=w17911:string)  [unwired: 1 in]
                        n3240 = Format Into String(format string="Where BREAKDOWN_DATE between '%s' and '%s' and  SHIFT_ID = '%d'  ", w17913, w17911, w17899) -> (resulting string=w17910:string)  [unwired: 2 in, 1 out]
                        n3241 = call <vilib>:"DB Tools Select Data.vi"("condition"=w17910, "error in (no error)"=w17919, "columns"=string[] ["BREAKDOWN_DATE"], "table"="STATION_1_LOG_HISTORY", "connection reference"=w17921) -> ("error out"=w17906:errorcluster, "data"=w17909:variant[][], "connection reference out"=w17920:T2)  [unwired: 1 in]
                        n3242 = property on="Table 2" class="Tbl (strict)"("Visible"=FALSE) -> ()  [unwired: 2 in, 2 out]
                        n3243 = xnode "Database Variant To Data"("database variant"=w17909, "error in (no error)"=w17906, "type"=string[][] [] ("Elements Found")) -> ("data"=w17907:string[][], "error out"=w17905:errorcluster)
                        n3244 = Index Array(array=w17907, index (col)=0 ("disabled index (col)")) -> (element=w17915:string[])  [unwired: 1 in]
                        n3245 = call "Search_1d_array_element.vi"("Count in"=string[] [] ("Elements Found"), "BD Date"=w17915, "Elements Found in"=string[] [] ("Elements Found")) -> ("Elements Found out"=w17902:string[])  [unwired: 4 in, 2 out]
                        n3246 = Build Array(w17902) -> (w17925:string[][])
                        n3247 = Transpose 2D Array(2D array=w17925) -> (transposed array=w17924:string[][])
                      }
                      frame #1 {
                        n3248 = disable-structure shown="Enabled" {
                          disable-tunnel: w17987 -> [w17998 w18000]
                          disable-tunnel: [w17997 w18000] -> w17986
                          disable-tunnel: w17985 -> [w17996 w18001]
                          disable-tunnel: [w17995 w18001] -> w17984
                          disable-tunnel: w17982 -> [w17993 _]
                          disable-tunnel: w17981 -> [w17992 _]
                          disable-tunnel: [w17991 _] -> w17980
                          disable-tunnel: [w17990 _] -> w17977
                          disable-tunnel: w17975 -> [w17989 _]
                          disable-tunnel: w17972 -> [w17988 w17999]
                          disable-tunnel: [_ w17999] -> w17971
                          frame Disabled {
                            n3249 = call "Stack_holderwise_total_bd_count_&_duration_2.vi"("Refnum in"=w17998, "BREAKDOWN_STK_HOLD_ID"=1, "condition"=w17989, "Form Date"=w17993, "To Date"=w17992, "error in (no error)"=w17996, "Shift"=w17988) -> ("Refnum out"=w17997:T2, "Count out"=w17991:string[], "appended array"=w17990:dbl[], "error out"=w17995:errorcluster)  [unwired: 5 in]
                          }
                          frame Enabled {
                          }
                        }
                        n3250 = call "NUMERIC TO STRING.vi"("appended array"=w17977) -> ("Array"=w17976:string[])  [unwired: 4 in]
                        n3251 = call "Insert_empty_element_with_zero.vi"("searched date"=w17980, "fixed date"=w17978) -> ("O/P"=w17973:string[])  [unwired: 9 in]
                        n3252 = call "Insert_empty_element_with_zero.vi"("searched date"=w17976, "fixed date"=w17978) -> ("O/P"=w17979:string[])  [unwired: 9 in]
                      }
                      frame #2 {
                        n3253 = disable-structure shown="Enabled" {
                          disable-tunnel: w18017 -> [w18031 w18033]
                          disable-tunnel: [w18030 w18033] -> w18016
                          disable-tunnel: w18015 -> [w18029 w18034]
                          disable-tunnel: [w18028 w18034] -> w18014
                          disable-tunnel: w18013 -> [w18027 _]
                          disable-tunnel: w18012 -> [w18026 _]
                          disable-tunnel: [w18025 _] -> w18011
                          disable-tunnel: [w18024 _] -> w18007
                          disable-tunnel: w18005 -> [w18023 _]
                          disable-tunnel: w18003 -> [w18021 w18032]
                          disable-tunnel: [_ w18032] -> w18002
                          frame Disabled {
                            n3254 = call "Stack_holderwise_total_bd_count_&_duration_2.vi"("Refnum in"=w18029, "BREAKDOWN_STK_HOLD_ID"=2, "condition"=w18023, "Form Date"=w18027, "To Date"=w18026, "error in (no error)"=w18031, "Shift"=w18021) -> ("Refnum out"=w18028:T2, "Count out"=w18025:string[], "appended array"=w18024:dbl[], "error out"=w18030:errorcluster)  [unwired: 5 in]
                          }
                          frame Enabled {
                          }
                        }
                        n3255 = call "Insert_empty_element_with_zero.vi"("searched date"=w18011, "fixed date"=w18008) -> ("O/P"=w18010:string[])  [unwired: 9 in]
                        n3256 = call "NUMERIC TO STRING.vi"("appended array"=w18007) -> ("Array"=w18006:string[])  [unwired: 4 in]
                        n3257 = call "Insert_empty_element_with_zero.vi"("searched date"=w18006, "fixed date"=w18008) -> ("O/P"=w18009:string[])  [unwired: 9 in]
                      }
                      frame #3 {
                        n3258 = disable-structure shown="Enabled" {
                          disable-tunnel: w18050 -> [w18066 w18068]
                          disable-tunnel: [w18065 w18068] -> w18049
                          disable-tunnel: w18048 -> [w18064 w18069]
                          disable-tunnel: [w18063 w18069] -> w18047
                          disable-tunnel: w18046 -> [w18062 _]
                          disable-tunnel: w18045 -> [w18061 _]
                          disable-tunnel: [w18060 _] -> w18044
                          disable-tunnel: [w18059 _] -> w18040
                          disable-tunnel: w18038 -> [w18058 _]
                          disable-tunnel: w18036 -> [w18056 w18067]
                          disable-tunnel: [_ w18067] -> w18035
                          frame Disabled {
                            n3259 = call "Stack_holderwise_total_bd_count_&_duration_2.vi"("Refnum in"=w18064, "BREAKDOWN_STK_HOLD_ID"=3, "condition"=w18058, "Form Date"=w18062, "To Date"=w18061, "error in (no error)"=w18066, "Shift"=w18056) -> ("Refnum out"=w18063:T2, "Count out"=w18060:string[], "appended array"=w18059:dbl[], "error out"=w18065:errorcluster)  [unwired: 5 in]
                          }
                          frame Enabled {
                          }
                        }
                        n3260 = call "Insert_empty_element_with_zero.vi"("searched date"=w18044, "fixed date"=w18041) -> ("O/P"=w18043:string[])  [unwired: 9 in]
                        n3261 = call "NUMERIC TO STRING.vi"("appended array"=w18040) -> ("Array"=w18039:string[])  [unwired: 4 in]
                        n3262 = call "Insert_empty_element_with_zero.vi"("searched date"=w18039, "fixed date"=w18041) -> ("O/P"=w18042:string[])  [unwired: 9 in]
                      }
                      frame #4 {
                        n3263 = disable-structure shown="Enabled" {
                          disable-tunnel: w18085 -> [w18103 w18106]
                          disable-tunnel: w18084 -> [w18102 w18105]
                          disable-tunnel: [w18101 w18105] -> w18083
                          disable-tunnel: [w18100 w18106] -> w18082
                          disable-tunnel: w18081 -> [w18099 _]
                          disable-tunnel: w18080 -> [w18098 _]
                          disable-tunnel: [w18097 _] -> w18079
                          disable-tunnel: [w18096 _] -> w18075
                          disable-tunnel: w18073 -> [w18095 _]
                          disable-tunnel: w18071 -> [w18093 w18104]
                          disable-tunnel: [_ w18104] -> w18070
                          frame Disabled {
                            n3264 = call "Stack_holderwise_total_bd_count_&_duration_2.vi"("Refnum in"=w18102, "BREAKDOWN_STK_HOLD_ID"=4, "condition"=w18095, "Form Date"=w18099, "To Date"=w18098, "error in (no error)"=w18103, "Shift"=w18093) -> ("Refnum out"=w18101:T2, "Count out"=w18097:string[], "appended array"=w18096:dbl[], "error out"=w18100:errorcluster)  [unwired: 5 in]
                          }
                          frame Enabled {
                          }
                        }
                        n3265 = call "Insert_empty_element_with_zero.vi"("searched date"=w18079, "fixed date"=w18076) -> ("O/P"=w18078:string[])  [unwired: 9 in]
                        n3266 = call "NUMERIC TO STRING.vi"("appended array"=w18075) -> ("Array"=w18074:string[])  [unwired: 4 in]
                        n3267 = call "Insert_empty_element_with_zero.vi"("searched date"=w18074, "fixed date"=w18076) -> ("O/P"=w18077:string[])  [unwired: 9 in]
                      }
                      frame #5 {
                        n3268 = call "Stack_holderwise_total_bd_count_&_duration_2.vi"("Refnum in"=w18120, "BREAKDOWN_STK_HOLD_ID"=5, "condition"=w18110, "Form Date"=w18117, "To Date"=w18118, "error in (no error)"=w18122, "Shift"=w18107) -> ("Refnum out"=w18119:T2, "Count out"=w18116:string[], "appended array"=w18112:dbl[], "error out"=w18121:errorcluster)  [unwired: 5 in]
                        n3269 = call "NUMERIC TO STRING.vi"("appended array"=w18112) -> ("Array"=w18111:string[])  [unwired: 4 in]
                        n3270 = call "Insert_empty_element_with_zero.vi"("searched date"=w18116, "fixed date"=w18114) -> ("O/P"=w18115:string[])  [unwired: 9 in]
                        n3271 = call "Insert_empty_element_with_zero.vi"("searched date"=w18111, "fixed date"=w18114) -> ("O/P"=w18113:string[])  [unwired: 9 in]
                      }
                      frame #6 {
                        n3272 = call "String to numeric.vi"("Array"=w18142) -> ("Array 2"=w18141:dbl[])  [unwired: 4 in]
                        n3273 = call "String to numeric.vi"("Array"=w18140) -> ("Array 2"=w18139:dbl[])  [unwired: 4 in]
                        n3274 = call "String to numeric.vi"("Array"=w18138) -> ("Array 2"=w18137:dbl[])  [unwired: 4 in]
                        n3275 = call "String to numeric.vi"("Array"=w18136) -> ("Array 2"=w18135:dbl[])  [unwired: 4 in]
                        n3276 = call "String to numeric.vi"("Array"=w18134) -> ("Array 2"=w18133:dbl[])  [unwired: 4 in]
                        n3277 = Decimal String To Number(string=w18147) -> (number=w18166:i32[])  [unwired: 2 in, 1 out]
                        n3278 = Decimal String To Number(string=w18148) -> (number=w18167:i32[])  [unwired: 2 in, 1 out]
                        n3279 = Decimal String To Number(string=w18149) -> (number=w18168:i32[])  [unwired: 2 in, 1 out]
                        n3280 = Decimal String To Number(string=w18150) -> (number=w18169:i32[])  [unwired: 2 in, 1 out]
                        n3281 = Decimal String To Number(string=w18151) -> (number=w18164:i32[])  [unwired: 2 in, 1 out]
                        n3282 = Compound Arithmetic op=ADD(w18141, w18139, w18137, w18135, w18133) -> (w18144:dbl[])
                        n3283 = Build Array(w18142) -> (w18163:string[][])
                        n3284 = Build Array(w18140) -> (w18162:string[][])
                        n3285 = Build Array(w18138) -> (w18161:string[][])
                        n3286 = Build Array(w18136) -> (w18160:string[][])
                        n3287 = Build Array(w18134) -> (w18159:string[][])
                        n3288 = Number To Fractional String(number=w18144, precision (6)=i16 2) -> (F-format string=w18143:string[])  [unwired: 2 in]
                        n3289 = Compound Arithmetic op=ADD(w18166, w18167, w18168, w18169, w18164) -> (w18170:i32[])
                        n3290 = Transpose 2D Array(2D array=w18163) -> (transposed array=w18157:string[][])
                        n3291 = Transpose 2D Array(2D array=w18162) -> (transposed array=w18156:string[][])
                        n3292 = Transpose 2D Array(2D array=w18161) -> (transposed array=w18155:string[][])
                        n3293 = Transpose 2D Array(2D array=w18160) -> (transposed array=w18154:string[][])
                        n3294 = Transpose 2D Array(2D array=w18159) -> (transposed array=w18153:string[][])
                        n3295 = Number To Decimal String(number=w18170) -> (decimal integer string=w18165:string[])  [unwired: 1 in]
                        n3296 = Build Array(w18143) -> (w18146:string[][])
                        n3297 = Transpose 2D Array(2D array=w18146) -> (transposed array=w18152:string[][])
                      }
                      frame #7 {
                        w18173 = string[] [""]
                        n3298 = Insert Into Array(array=w18183, index (col)=1 ("disabled index (col)"), new element #1=w18173, new element #2=w18173, new element #3=w18173, new element #4=w18173, new element #5=w18173, new element #6=w18173, new element #7=w18173, new element #8=w18173, new element #9=w18174, new element #10=w18175, new element #11=w18176, new element #12=w18177) -> (w18179:string[][])  [unwired: 1 in]
                        n3299 = call "flot graph for month n year.vi"("BD Date"=w18180, "error in (no error)"=w18182, "Count total"=w18176) -> ("error out"=w18181:errorcluster, "Run-Time Status"=w18178:cluster{"Array 2":timestamp[], dbl[]})  [unwired: 7 in]
                        n3300 = local write "Run-Time Status"(w18178) -> ()
                        n3301 = local write "Table"(w18179) -> ()
                      }
                    }
                  }
                  frame "all" {
                  }
                }
              }
            }
          }
        }
      }
    }
    n3302 = disable-structure shown="Enabled" {
      frame Disabled {
        n3303 = local read "Form Date"() -> (w113:timestamp)
        n3304 = local read "Select Station"() -> (w111:string)
        n3305 = local read "To Date"() -> (w112:timestamp)
        n3306 = local read "Shift"() -> (w95:string)
        n3307 = call "Condition _string_4_prod_count_month.vi"("From Date"=w113, "Select Stakeholder"=w111, "To Date"=w112, "Shift"=w95) -> ()  [unwired: 4 in, 8 out]
        n3308 = case shown="\"ALL\", Default" w95 {
          tunnel: _ -> [_ w119 w122 w127 w132 w137 w142 w147]
          tunnel: [w114 w115 w121 w126 w131 w136 w141 w146] -> w105
          tunnel: [w114 w116 w120 w126 w131 w136 w141 w146] -> w104
          tunnel: [w114 w116 w121 w125 w131 w136 w141 w146] -> w103
          tunnel: [w114 w116 w121 w126 w130 w136 w141 w146] -> w102
          tunnel: [w114 w116 w121 w126 w131 w135 w141 w146] -> w101
          tunnel: [_ w116 w121 w126 w131 w136 w140 w146] -> w97
          tunnel: [_ w116 w121 w126 w131 w136 w141 w145] -> w96
          tunnel: _ -> [_ w115 w120 w125 w130 w135 w140 w145]
          frame "False" {
            w114 = string[] ["0"]
          }
          frame "ALL", Default {
            n3309 = Array Size(array=w119) -> (size(s)=w118:i32)
            n3310 = Number To Decimal String(number=w119) -> ()  [unwired: 1 in, 1 out]
            n3311 = Initialize Array("0", w118) -> (w116:string[])
          }
          frame "ST 1" {
            (unwired) string[] ["0"]
            n3312 = Array Size(array=w122) -> (size(s)=w124:i32)
            n3313 = Number To Decimal String(number=w122) -> ()  [unwired: 1 in, 1 out]
            n3314 = Initialize Array("0", w124) -> (w121:string[])
          }
          frame "ST 2" {
            (unwired) string[] ["0"]
            n3315 = Array Size(array=w127) -> (size(s)=w129:i32)
            n3316 = Number To Decimal String(number=w127) -> ()  [unwired: 1 in, 1 out]
            n3317 = Initialize Array("0", w129) -> (w126:string[])
          }
          frame "ST 3" {
            (unwired) string[] ["0"]
            n3318 = Array Size(array=w132) -> (size(s)=w134:i32)
            n3319 = Number To Decimal String(number=w132) -> ()  [unwired: 1 in, 1 out]
            n3320 = Initialize Array("0", w134) -> (w131:string[])
          }
          frame "ST 4" {
            (unwired) string[] ["0"]
            n3321 = Array Size(array=w137) -> (size(s)=w139:i32)
            n3322 = Number To Decimal String(number=w137) -> ()  [unwired: 1 in, 1 out]
            n3323 = Initialize Array("0", w139) -> (w136:string[])
          }
          frame "ST 5" {
            (unwired) string[] ["0"]
            n3324 = Array Size(array=w142) -> (size(s)=w144:i32)
            n3325 = Number To Decimal String(number=w142) -> ()  [unwired: 1 in, 1 out]
            n3326 = Initialize Array("0", w144) -> (w141:string[])
          }
          frame "ST 6" {
            (unwired) string[] ["0"]
            n3327 = Array Size(array=w147) -> (size(s)=w149:i32)
            n3328 = Number To Decimal String(number=w147) -> ()  [unwired: 1 in, 1 out]
            n3329 = Initialize Array("0", w149) -> (w146:string[])
          }
        }
        n3330 = Decimal String To Number(string=w105) -> (number=w106:i32[])  [unwired: 2 in, 1 out]
        n3331 = Decimal String To Number(string=w104) -> (number=w107:i32[])  [unwired: 2 in, 1 out]
        n3332 = Decimal String To Number(string=w103) -> (number=w108:i32[])  [unwired: 2 in, 1 out]
        n3333 = Decimal String To Number(string=w102) -> (number=w109:i32[])  [unwired: 2 in, 1 out]
        n3334 = Decimal String To Number(string=w101) -> (number=w100:i32[])  [unwired: 2 in, 1 out]
        n3335 = Compound Arithmetic op=ADD(w106, w107, w108, w109, w100) -> (w110:i32[])
        n3336 = Number To Decimal String(number=w110) -> (decimal integer string=w98:string[])  [unwired: 1 in]
        n3337 = Build Array(w105, w104, w103, w102, w101, w97, w96, w98) -> (w99:string[])  [unwired: 1 out]
      }
      frame Enabled {
      }
    }
  }
  n3338 = call <vilib>:"DB Tools Close Connection.vi"("error in (no error)"=w16, "connection reference"=w15) -> ("error out"=w18:errorcluster)  [unwired: 5 in]
  n3339 = call <vilib>:"Clear Errors.vi"("error in (no error)"=w18) -> ("error out"=w17:errorcluster)  [unwired: 5 in, 1 out]
  n3340 = property class="App"(error in=w17) -> (error out=w20:errorcluster, "App.Kind"=w21:T3)  [unwired: 1 in, 1 out]
  n3341 = case shown="Default" w21 {
    tunnel: w20 -> [w18187 w18189]
    tunnel: [w18186 w18188] -> w19
    frame Default {
      n3342 = invoke class="VI" method="FP.Close"(error in=w18187) -> (error out=w18186:errorcluster)  [unwired: 2 in, 2 out]
    }
    frame "Run Time System" {
      n3343 = invoke class="VI" method="FP.Close"(error in=w18189) -> (error out=w18188:errorcluster)  [unwired: 2 in, 2 out]
    }
  }
  "error out" <- w19
